vi "Pre Launch Init.vi"(11 "Threshold in":refnum<class "Threshold.lvclass">) -> (0 "error out":errorcluster, 3 "Threshold out":refnum<class "Threshold.lvclass">)   [LabVIEW 2016, in "Tests.lvlib" / "Threshold.lvclass"]
doc: "Creates neccessary user events for threshold actor."
uses:
  Threshold.lvclass
  <vilib>/vision/Image Controls.llb/IMAQ Image.ctl
  Threshold.lvclass/Threshold.ctl
  Tests.lvclass
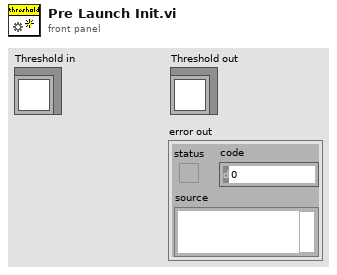
[diagram p1: front panel]
types:
  T1 = typedef "IMAQ Image.ctl" = refnum<image>
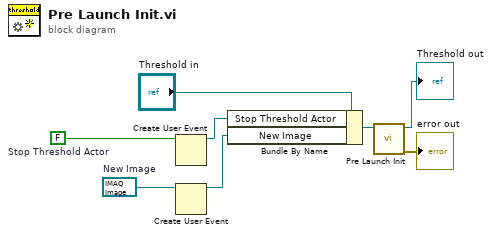
[diagram p0: block diagram]
diagram:
  w5 = T1 refnum  # New Image
  w6 = FALSE  # Stop Threshold Actor
  n1 = Create User Event(user event datatype=w6) -> (user event=w2:refnum<user-event>)  [unwired: 1 in, 1 out]
  n2 = Create User Event(user event datatype=w5) -> (user event=w1:refnum<user-event>)  [unwired: 1 in, 1 out]
  n3 = Bundle By Name(cluster="Threshold in", "Stop Threshold Actor"=w2, "New Image"=w1) -> (w3:refnum<class "Threshold.lvclass">)
  n4 = call-parent "Pre Launch Init.vi"("Actor in"=w3) -> ("error out"=→"error out":errorcluster, "Actor out"=→"Threshold out":refnum<class "Threshold.lvclass">)  [unwired: 9 in]
